vi "read all lines.vi"(8 "error in (no error)":errorcluster, 11 "USB-6000 in":refnum<class "USB-6000.lvclass">) -> (0 "error out":errorcluster, 2 "Array":dbl[](array[numeric]), 3 "USB-6000 out":refnum<class "USB-6000.lvclass">)   [LabVIEW 2025, in "USB IO.lvlib" / "USB-6000.lvclass"]
uses:
  USB-6000.lvclass
  USB-6000.lvclass/USB-6000.ctl
  <vilib>/DAQmx/read.llb/DAQmx Read (Analog DBL 1Chan 1Samp).vi
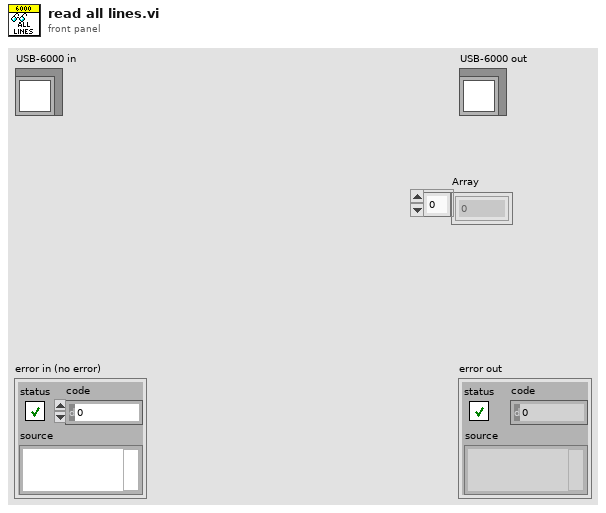
[diagram p1: front panel]
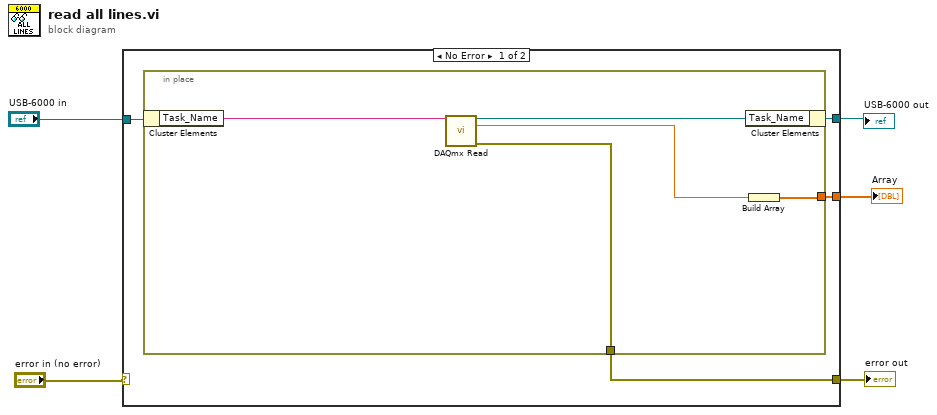
[diagram p0: block diagram]
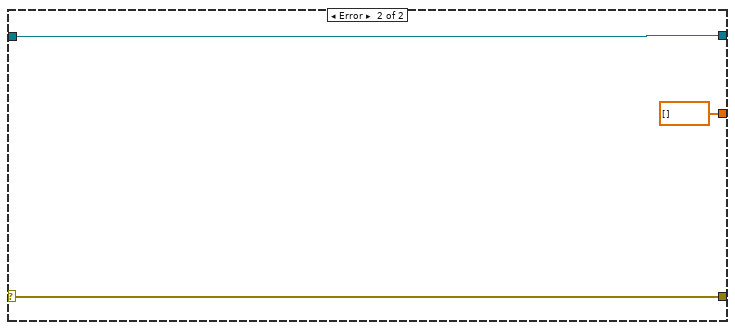
[diagram p2: hidden frame]
diagram:
  n1 = case shown="No Error" "error in (no error)" {
    selector: "error in (no error)" -> [_ w16]
    tunnel: [w7 w16] -> w4
    tunnel: "USB-6000 in" -> [w9 w17]
    tunnel: [w8 w17] -> w2
    tunnel: [w6 dbl[] [] ("data")] -> w1
    frame No Error {
      n2 = in-place {
        in-place-border: [w12] -> w7
        in-place-border: [w11] -> w6
        n3 = in-place-cluster #1(w9) -> ("Task_Name"=w14:string)
        n4 = call-poly <vilib>:"DAQmx Read.vi"("task/channels in"=w14) -> ("task out"=w13:refnum<k21>, "data"=w10:dbl, "error out"=w12:errorcluster)  [unwired: 12 in]
        n5 = in-place-cluster #1("Task_Name"=w13) -> (w8:refnum<class "USB-6000.lvclass">)
        n6 = Build Array(w10) -> (w11:dbl[])
      }
    }
    frame Error {
    }
  }
  "error out" <- w4
  "USB-6000 out" <- w2
  "Array" <- w1
